vi "PID_2Chan_V4_1loop_multiTs.vi"() -> ()   [LabVIEW 2016]
uses:
  <vilib>/addons/control/pid/pid.llb/PID Advanced (DBL Array).vi
  <vilib>/addons/control/pid/pid.llb/PID Parameter Manager (DBL Array).vi
  <vilib>/addons/control/pid/pid.llb/PID Derivative Action Buffered (DBL Array).vi
  <vilib>/addons/control/pid/pid.llb/PID Get Advanced Error (DBL Array).vi
  <vilib>/addons/control/pid/pid.llb/PID Integral Action Buffered (DBL Array).vi
  <vilib>/addons/control/pid/pid.llb/PID Resize 1D Array.vi
  <vilib>/addons/control/pid/pid.llb/PID Get Advanced Error (DBL).vi
  <userlib>/Fluigent/Fluigent MFCS/FluigentMFCS_Full.llb/MFCS_EZ Detect.vi
  <userlib>/Fluigent/Fluigent MFCS/FluigentMFCS_Full.llb/MFCS_EZ Initialization.vi
  <userlib>/Fluigent/Fluigent MFCS/FluigentMFCS_Full.llb/MFCS_EZ Write Channel Pressure.vi
  Globals/PressuresGlobal.vi
  <userlib>/Fluigent/Fluigent MFCS/FluigentMFCS_Full.llb/MFCS_EZ Close.vi
  <vilib>/addons/control/pid/NI_PID_pid.lvlib
  <vilib>/Analysis/NI_AALBase.lvlib
  <vilib>/Analysis/baseanly.llb/Mean (DBL).vi
panel:
  in  "Total Odor Flow":dbl=425.0
  in  "Ftot Setpoint":dbl=531.25
  in  "AutoControl PID":bool
  out "Pressure Stable?":bool=TRUE
  in  "Ftot Stability Threshold 2":dbl=0.631165
  in  "F1 Stability Threshold":dbl=0.631165
  out "Setpoint Reached?":bool
  in  "Pressure Resolution":dbl=0.631165
  in  "Control Pressure":dbl format="%_6g"
  in  "Control Pressure Channel":i16
  in  "output cluster":T1
  out "Set Pressure":dbl[](array[numeric])=[924.5131355020292, 768.8474129854441] format="%_10g"
  in  "linearity":dbl[](array[numeric])=[0.30000000000000004, 0.4] format="%.2f"
  out "Flow 1 plot 2":cluster{"[0]":dbl, "[1]":dbl}(graph)={"[0]"=425.0, "[1]"=424.3360907434235}
  out "Flow Rates":dbl[](array[numeric])=[382.62235422818463, 424.3360907434235]
  in  "FTot PID gains":cluster{"P":dbl, "I":dbl, "D":dbl}={"P"=0.02, "I"=0.0, "D"=0.0} {"D" format="%.3f"; "I" format="%.3f"; "P" format="%.5f"}
  in  "Vals to display":dbl=1235.0
  out "Flow 1 plot":cluster{"[0]":dbl, "[1]":dbl}(graph)={"[0]"=382.62235422818463, "[1]"=382.5}
  out "Ferr":T2(graph)={"output[0]"=0.005169696367242157, "output[1]"=0.005463430350005343, "output[2]"=0.0}
  out "Pressures":dbl[](array[numeric])=[924.6800537109375, 768.7783813476562]
  in  "F1 PID gains":cluster{"P":dbl, "I":dbl, "D":dbl}={"P"=0.004, "I"=0.0, "D"=0.0} {"D" format="%.3f"; "I" format="%.3f"; "P" format="%.5f"}
  in  "reset Averging":bool
  in  "Set current Pressure\n to manual pressure":bool=TRUE
  out "Pressures":T3(graph)={"[0]"=924.6800537109375, "[1]"=768.7783813476562, "[2]"=924.5131355020292, "[3]"=768.8474129854441}
  in  "stop":bool=TRUE
  in  "Control Valves":enum16{"1", "2", "3", "4", "5", "6", "7", "8"}[](array[ring])=[enum."7", enum."8"]
  in  "Pressure Channels":i16[](array[numeric])=[2, 1]
  in  "Manual Pressure Set":dbl[](array[numeric])=[924.5131355020292, 768.8474129854441] format="%_6g"
  in  "reinitialize? (F)":bool
  in  "Add Ctrl?":bool
  in  "Boards":enum16{"A", "B", "C"}[](array[ring])=[enum."A", enum."A"]
  in  "Valves":enum16{"1", "2", "3", "4", "5", "6", "7", "8"}[](array[ring])=[enum."5", enum."7"]
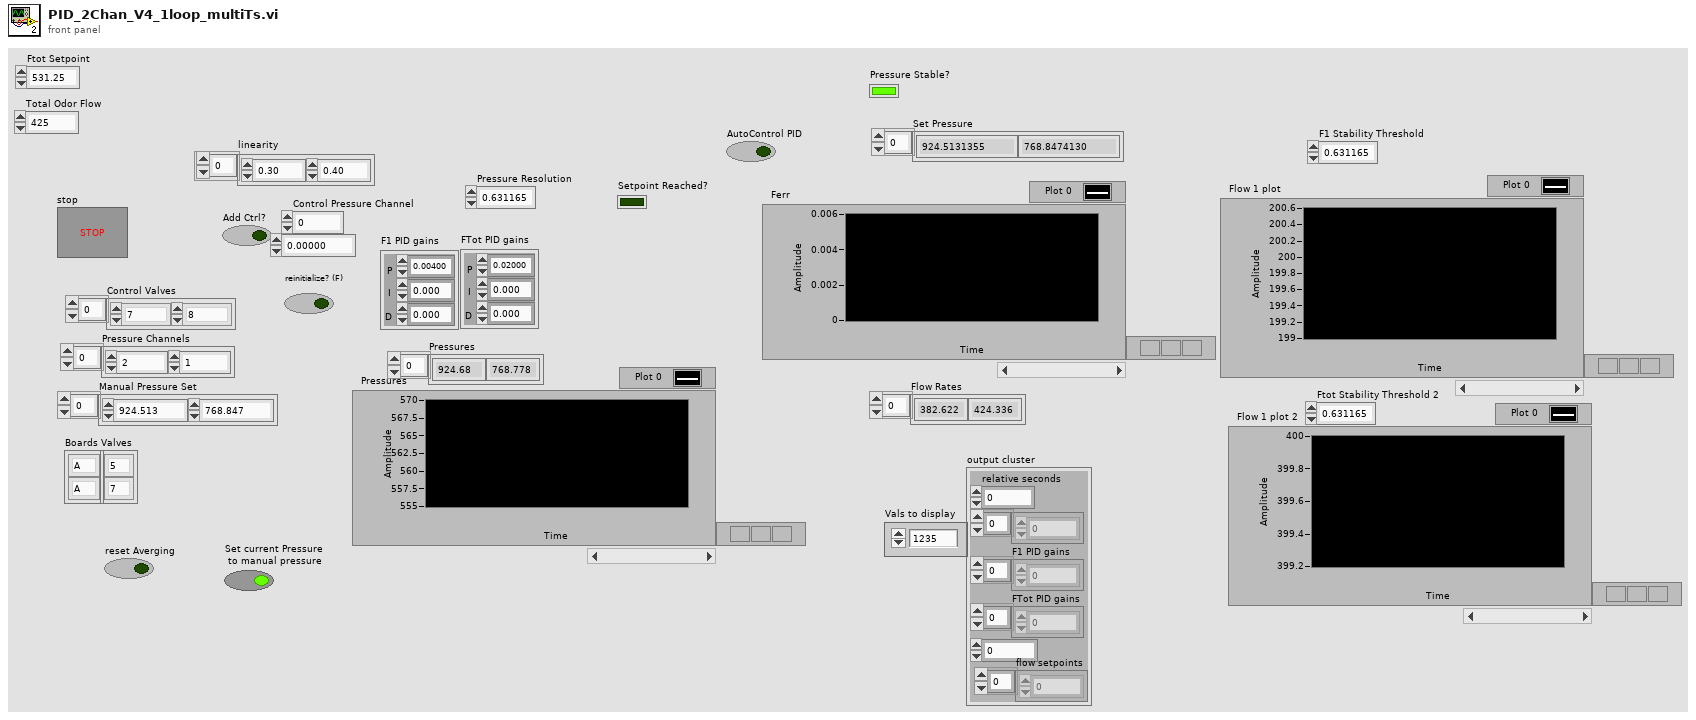
[diagram p1: front panel]
types:
  T1 = cluster{"relative seconds":dbl, "Pressures":dbl[], "F1 PID gains":dbl[], "FTot PID gains":dbl[], "PID On?":i16, "flow setpoints":dbl[]}
  T2 = cluster{"output[0]":dbl, "output[1]":dbl, "output[2]":dbl}
  T3 = cluster{"[0]":dbl, "[1]":dbl, "[2]":dbl, "[3]":dbl}
  T4 = cluster{"setpoint high":dbl, "setpoint low":dbl}[]
  T5 = typedef "_EZmfcsSN.ctl" = u16
  T6 = typedef "_EZmfcsRefNum.ctl" = refnum<k1>
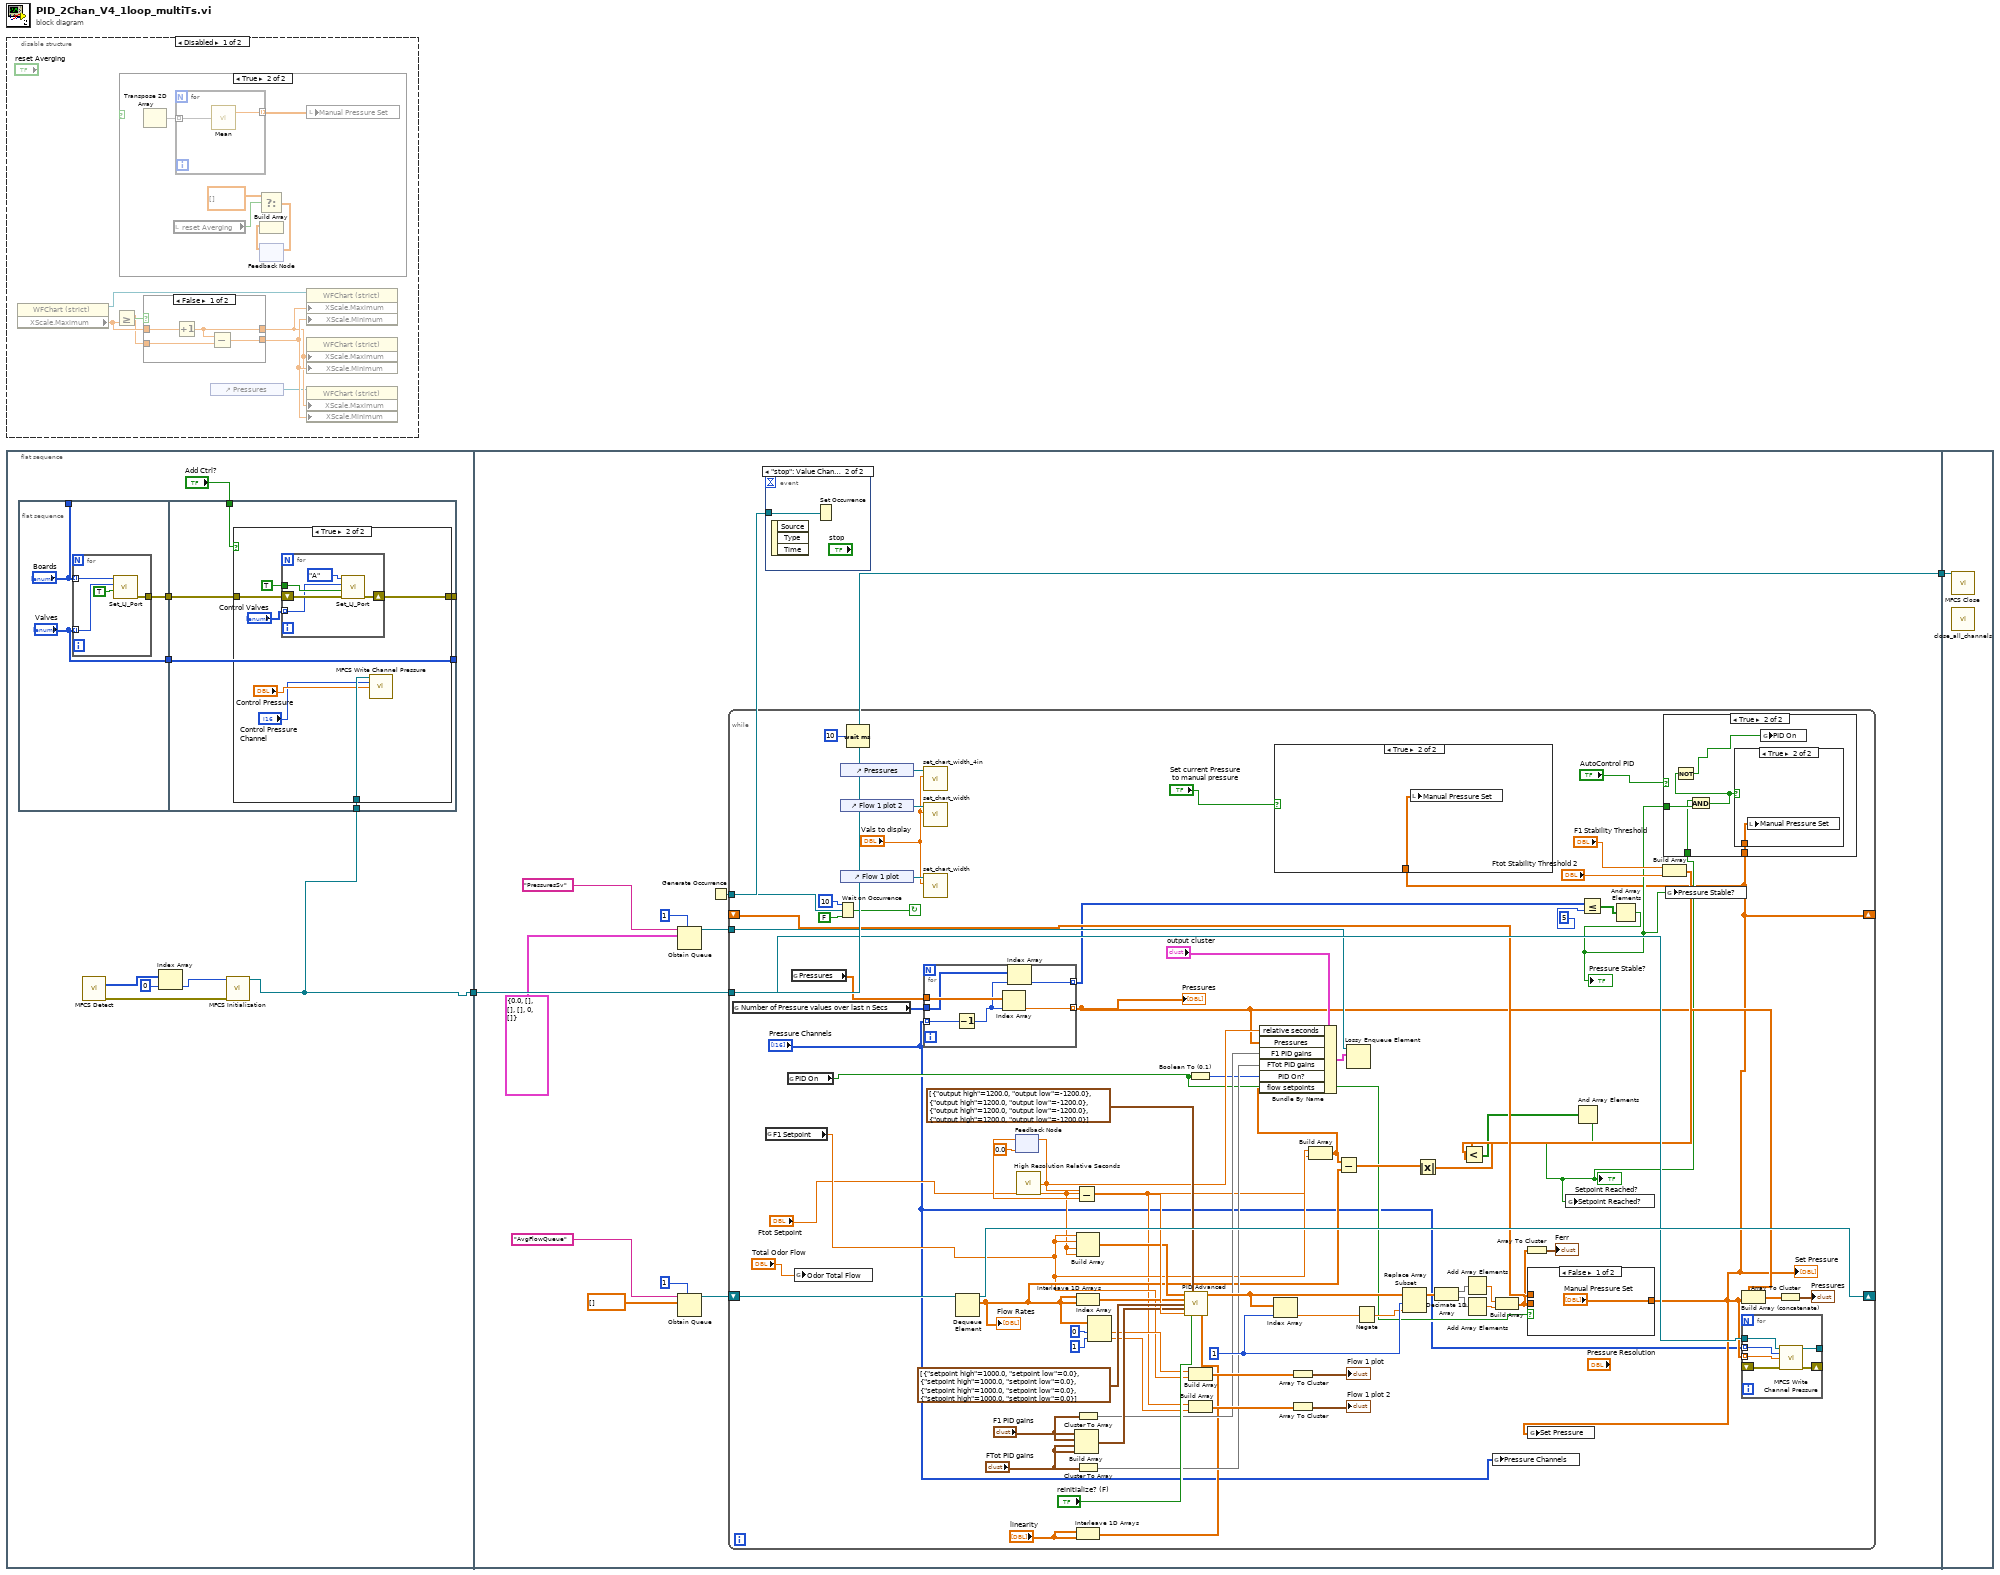
[diagram p0: block diagram]
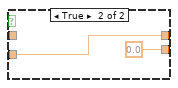
[diagram p2: hidden frame]
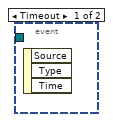
[diagram p6: hidden frame]
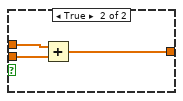
[diagram p10: hidden frame]
diagram:
  n1 = disable-structure shown="Disabled" {
    frame Disabled {
      n2 = property on="Property Node" class="WFChart (strict)"() -> (reference=w6:refnum<vi>, reference out=w7:refnum<vi>, "XScale.Maximum"=w5:dbl)  [unwired: 1 in, 1 out]
      n3 = Greater Or Equal?(y=w5) -> (x=w3:dbl, x >= y?=w4:bool)
      n4 = case shown="True" w12 {
        frame False {
        }
        frame True {
          n5 = Transpose 2D Array() -> (transposed array=w22:dbl[][])  [unwired: 1 in]
          n6 = local read "reset Averging"() -> (w23:bool)
          n7 = for {
            tunnel: w22 -> [w26] mode=indexing
            tunnel: [w25] -> w19 mode=indexing
            n8 = call-poly <vilib>:"Mean.vi"("X"=w26) -> ("mean"=w25:dbl)  [unwired: 1 out]
          }
          n9 = Select(t=dbl[][] [] ("appended array"), s=w23) -> (s? t:f=w20:dbl[][])  [unwired: 1 in]
          n10 = feedback-in #1(w20) -> ()
          n11 = feedback #1() -> (w24:dbl[][])  [unwired: 1 in]
          n12 = Build Array(w24) -> ()  [unwired: 1 in, 1 out]
          n13 = local write "Manual Pressure Set"(w19) -> ()
        }
      }
      n14 = case shown="False" w4 {
        tunnel: w3 -> [w14 w18]
        tunnel: w5 -> [w16 _]
        tunnel: [w13 w18] -> w10
        tunnel: [w15 0.0] -> w11
        frame False {
          n15 = Increment(x=w16) -> (x+1=w13:dbl)
          n16 = Subtract(x=w13, y=w14) -> (x-y=w15:dbl)
        }
        frame True {
        }
      }
      n17 = control-ref of="Pressures"() -> (w8:refnum<vi>)
      n18 = property on="Property Node" class="WFChart (strict)"(reference=w7, "XScale.Maximum"=w10, "XScale.Minimum"=w11) -> ()  [unwired: 1 in, 2 out]
      n19 = property on="Property Node" class="WFChart (strict)"("XScale.Maximum"=w10, "XScale.Minimum"=w11) -> (reference=w9:refnum<vi>)  [unwired: 1 in, 2 out]
      n20 = property on="Property Node" class="WFChart (strict)"(reference=w8, "XScale.Maximum"=w10, "XScale.Minimum"=w11) -> ()  [unwired: 1 in, 2 out]
    }
    frame Enabled {
    }
  }
  n21 = flat-sequence {
    tunnel: [w27] -> w1
    tunnel: [w61] -> w2
    tunnel: w1 -> [w61]
    tunnel: w2 -> [w172]
    frame #0 {
      n22 = flat-sequence {
        tunnel: ["Boards"] -> _
        tunnel: [w37] -> w34
        tunnel: ["Valves"] -> w33
        tunnel: [w46] -> _
        tunnel: [w44] -> _
        tunnel: w34 -> [w45]
        tunnel: w33 -> [w46]
        tunnel: "Add Ctrl?" -> [w43]
        tunnel: w27 -> [w42]
        frame #0 {
          n23 = for {
            tunnel: "Valves" -> [w41] mode=indexing
            tunnel: "Boards" -> [w40] mode=indexing
            tunnel: [w38] -> w37
            n24 = call "Set_LJ_Port.vi"("State"=TRUE, "Channel"=w41, "Flowboard"=w40) -> ("error out"=w38:errorcluster)  [unwired: 8 in]
          }
        }
        frame #1 {
          n25 = case shown="True" w43 {
            tunnel: w45 -> [w47 w54]
            tunnel: [w47 w53] -> w44
            tunnel: w42 -> [_ w50]
            frame False {
            }
            frame True {
              n26 = for {
                tunnel: TRUE ("State") -> [w57]
                shift-right: [w58] -> w53
                shift-left: w54 -> [w59]
                tunnel: "Control Valves" -> [w56] mode=indexing
                n27 = call "Set_LJ_Port.vi"("error in"=w59, "State"=w57, "Channel"=w56, "Flowboard"=enum16{"A", "B", "C"}."A") -> ("error out"=w58:errorcluster)  [unwired: 7 in]
              }
              n28 = call-poly <userlib>:"MFCS Write Channel Pressure.vi"("MFCS_EZ"=w50, "Channel Number (default=1)"="Control Pressure Channel", "Pressure (mBar)"="Control Pressure") -> ()  [unwired: 11 in, 2 out]
            }
          }
        }
      }
      n29 = call-poly <userlib>:"MFCS Detect.vi"() -> ("[SN MFCS_EZ]"=w28:T5[], "error out"=w30:errorcluster)  [unwired: 14 in]
      n30 = Index Array(array=w28, index=0) -> (element=w29:T5)
      n31 = call-poly <userlib>:"MFCS Initialization.vi"("SN MFCS_EZ"=w29, "error in (no error)"=w30) -> ("MFCS_EZ"=w27:T6)  [unwired: 11 in, 2 out]
    }
    frame #1 {
      n32 = Obtain Queue(max queue size (-1, unlimited)=1, name (unnamed)="PressuresSv", element data type=T1 {"relative seconds"=0.0, "Pressures"=[], "F1 PID gains"=[], "FTot PID gains"=[], "PID On?"=0, "flow setpoints"=[]} ("output cluster")) -> (queue out=w63:refnum<queue>)  [unwired: 2 in, 2 out]
      n33 = Obtain Queue(max queue size (-1, unlimited)=1, name (unnamed)="AvgFlowQueue", element data type=dbl[] [] ("appended array")) -> (queue out=w67:refnum<queue>)  [unwired: 2 in, 2 out]
      n34 = Generate Occurrence() -> (w66:refnum<k4>)
      n35 = while {
        shift-right: [w147] -> _
        shift-left: w67 -> [w148]
        tunnel: w66 -> [w133]
        tunnel: w61 -> [w122]
        shift-right: [w72] -> _
        shift-left: _ -> [w119]
        tunnel: w63 -> [w111]
        stop <- w132 continue-if-true
        w140 = 1 ("index")
        n36 = global read "PressuresGlobal.vi" "Number of Pressure values over last n Secs"() -> (w92:i32[])
        n37 = global read "PressuresGlobal.vi" "F1 Setpoint"() -> (w78:dbl)
        n38 = global read "PressuresGlobal.vi" "PID On"() -> (w77:bool)
        n39 = global read "PressuresGlobal.vi" "Pressures"() -> (w93:dbl[])
        n40 = global write "PressuresGlobal.vi" "Odor Total Flow"("Total Odor Flow") -> ()
        n41 = Wait on Occurrence(1:FALSE ("ignore previous (T)"), 2:w133, 3:10 ("ms timeout (-1)")) -> (0:w132:bool)
        n42 = control-ref of="Pressures"() -> (w121:refnum<vi>)
        n43 = control-ref of="Flow 1 plot 2"() -> (w105:refnum<vi>)
        n44 = control-ref of="Flow 1 plot"() -> (w104:refnum<vi>)
        n45 = Wait (ms)(milliseconds to wait=u32 10) -> ()  [unwired: 1 out]
        n46 = call "set_chart_width_4in.vi"("Values to Display"="Vals to display", "Ref In"=w121) -> ()  [unwired: 10 in]
        n47 = call "set_chart_width.vi"("Values to Display"="Vals to display", "Ctl Refnum"=w105) -> ()  [unwired: 10 in]
        n48 = call "set_chart_width.vi"("Values to Display"="Vals to display", "Ctl Refnum"=w104) -> ()  [unwired: 10 in]
        n49 = for {
          tunnel: "Pressure Channels" -> [w160] mode=indexing
          tunnel: w93 -> [w161]
          tunnel: [w159] -> w81 mode=indexing
          tunnel: w92 -> [w158]
          tunnel: [w156] -> w91 mode=indexing
          n50 = Decrement(x=w160) -> (x-1=w157:i16)
          n51 = Index Array(array=w161, index=w157) -> (element=w159:dbl)
          n52 = Index Array(array=w158, index=w157) -> (element=w156:i32)
        }
        "Pressures" <- w81
        n53 = Dequeue Element(queue=w148) -> (queue out=w147:refnum<queue>, element=w89:dbl[])  [unwired: 2 in, 2 out]
        "Flow Rates" <- w89
        n54 = feedback #2(0.0 ("relative seconds")) -> (w143:dbl)
        n55 = call <vilib>:"High Resolution Relative Seconds.vi"() -> ("relative seconds"=w110:dbl)
        n56 = feedback-in #2(w110) -> ()
        n57 = Subtract(x=w110, y=w143) -> (x-y=w142:dbl)
        n58 = Build Array("F1 PID gains", "F1 PID gains", "FTot PID gains", "FTot PID gains") -> (w136:cluster{"P":dbl, "I":dbl, "D":dbl}[])
        n59 = Build Array(w78, w78, "Ftot Setpoint", "Ftot Setpoint") -> (w130:dbl[])
        n60 = Interleave 1D Arrays(w89, w89) -> (w124:dbl[])
        n61 = Cluster To Array(cluster="F1 PID gains") -> (array=w109:dbl[])
        n62 = Cluster To Array(cluster="FTot PID gains") -> (array=w108:dbl[])
        n63 = Interleave 1D Arrays("linearity", "linearity") -> (w97:dbl[])
        n64 = Index Array(array=w89, index #1=0 ("index"), index #2=1 ("index")) -> (element #1=w102:dbl, element #2=w101:dbl)
        n65 = call-poly <vilib>:"PID Advanced.vi"("setpoint"=w130, "output range"=cluster{"output high":dbl, "output low":dbl}[] [{"output high"=1200.0, "output low"=-1200.0}, {"output high"=1200.0, "output low"=-1200.0}, {"output high"=1200.0, "output low"=-1200.0}, {"output high"=1200.0, "output low"=-1200.0}], "process variable"=w124, "setpoint range"=T4 [{"setpoint high"=1000.0, "setpoint low"=0.0}, {"setpoint high"=1000.0, "setpoint low"=0.0}, {"setpoint high"=1000.0, "setpoint low"=0.0}, {"setpoint high"=1000.0, "setpoint low"=0.0}], "PID gains"=w136, "dt (s)"=w142, "reinitialize? (F)"="reinitialize? (F)", "linearity"=w97) -> ("output"=w137:dbl[])  [unwired: 6 in, 1 out]
        n66 = Boolean To (0,1)(Boolean=w77) -> (0, 1=w107:i16)
        n67 = Build Array(w102, w78) -> (w115:dbl[])
        n68 = Build Array("Ftot Setpoint", w101) -> (w113:dbl[])
        n69 = Index Array(array=w137, index=w140) -> (element=w139:dbl)
        n70 = Array To Cluster(array=w115) -> (cluster=→"Flow 1 plot":cluster{"[0]":dbl, "[1]":dbl})
        n71 = Array To Cluster(array=w113) -> (cluster=→"Flow 1 plot 2":cluster{"[0]":dbl, "[1]":dbl})
        n72 = Build Array(w78, "Ftot Setpoint") -> (w79:dbl[])
        n73 = Bundle By Name(cluster="output cluster", "relative seconds"=w110, "Pressures"=w81, "F1 PID gains"=w109, "FTot PID gains"=w108, "PID On?"=w107, "flow setpoints"=w79) -> (w95:T1)
        n74 = Subtract(x=w79, y=w89) -> (x-y=w88:dbl[])
        n75 = Lossy Enqueue Element(queue=w111, element=w95) -> ()  [unwired: 1 in, 4 out]
        n76 = Negate(x=w139) -> (-x=w138:dbl)
        n77 = Replace Array Subset(array=w137, new element=w138, index=w140) -> (w129:dbl[])
        n78 = Absolute Value(x=w88) -> (abs(x)=w84:dbl[])
        n79 = Decimate 1D Array(w129) -> (w128:dbl[], w127:dbl[])
        n80 = Add Array Elements(numeric array=w128) -> (sum=w126:dbl)
        n81 = Add Array Elements(numeric array=w127) -> (sum=w125:dbl)
        n82 = global write "PressuresGlobal.vi" "Pressure Channels"("Pressure Channels") -> ()
        n83 = Build Array(w126, w125) -> (w118:dbl[])
        n84 = Array To Cluster(array=w118) -> (cluster=→"Ferr":cluster{"[0]":dbl, "[1]":dbl, "[2]":dbl})
        n85 = case shown="False" w77 {
          tunnel: w118 -> [_ w171]
          tunnel: w119 -> [_ w170]
          tunnel: ["Manual Pressure Set" w169] -> w72
          frame False {
          }
          frame True {
            n86 = Add(x=w170, y=w171) -> (x+y=w169:dbl[])
          }
        }
        "Set Pressure" <- w72
        n87 = case shown="True" "Set current Pressure\n to manual pressure" {
          tunnel: w72 -> [_ w155]
          frame False {
          }
          frame True {
            n88 = local write "Manual Pressure Set"(w155) -> ()
          }
        }
        n89 = global write "PressuresGlobal.vi" "Set Pressure"(w72) -> ()
        n90 = Less Or Equal?(x=w91, y=5) -> (x <= y?=w82:bool[])
        n91 = And Array Elements(Boolean array=w82) -> (logical AND=w73:bool)
        "Pressure Stable?" <- w73
        n92 = Build Array("F1 Stability Threshold", "Ftot Stability Threshold 2") -> (w85:dbl[])
        n93 = Less?(x=w84, y=w85) -> (x < y?=w83:bool[])
        n94 = And Array Elements(Boolean array=w83) -> (logical AND=w74:bool)
        "Setpoint Reached?" <- w74
        n95 = global write "PressuresGlobal.vi" "Setpoint Reached?"(w74) -> ()
        n96 = case shown="True" "AutoControl PID" {
          tunnel: w73 -> [_ w153]
          tunnel: w74 -> [_ w152]
          tunnel: w72 -> [_ w151]
          frame False {
          }
          frame True {
            n97 = And(x=w152, y=w153) -> (x .and. y?=w150:bool)
            n98 = Not(x=w150) -> (.not. x?=w149:bool)
            n99 = case shown="True" w150 {
              tunnel: w151 -> [_ w154]
              frame False {
              }
              frame True {
                n100 = local write "Manual Pressure Set"(w154) -> ()
              }
            }
            n101 = global write "PressuresGlobal.vi" "PID On"(w149) -> ()
          }
        }
        n102 = global write "PressuresGlobal.vi" "Pressure Stable?"(w73) -> ()
        n103 = Build Array (concatenate)(w81, w72) -> (w106:dbl[])
        n104 = for {
          shift-right: [w166] -> _
          shift-left: _ -> [w167]
          tunnel: [w165] -> _
          tunnel: "Pressure Channels" -> [w164] mode=indexing
          tunnel: w72 -> [w163] mode=indexing
          tunnel: w122 -> [w162]
          n105 = call-poly <userlib>:"MFCS Write Channel Pressure.vi"("MFCS_EZ"=w162, "Channel Number (default=1)"=w164, "Pressure (mBar)"=w163, "error in (no error)"=w167) -> ("MFCS_EZ out"=w165:T6, "error out"=w166:errorcluster)  [unwired: 10 in]
        }
        n106 = Array To Cluster(array=w106) -> (cluster=→"Pressures":T3)
      }
      n107 = event shown="[1] \"stop\": Value Change" {
        selector: _ -> [_ _]
        dyn-events: _ -> [_ _]
        timeout: _ -> [_ _]
        tunnel: w66 -> [_ w70]
        event Timeout {
          n108 = event-data() -> ()  [unwired: 1 in, 3 out]
        }
        event "stop": Value Change {
          n109 = event-data() -> ()  [unwired: 1 in, 3 out]
          n110 = Set Occurrence(w70) -> ()
        }
      }
    }
    frame #2 {
      n111 = call-poly <userlib>:"MFCS Close.vi"("MFCS_EZ"=w172) -> ()  [unwired: 14 in, 1 out]
      n112 = call "close_all_channels.vi"() -> ()  [unwired: 12 in]
    }
  }
